vi "Configure Chart.vi"(8 "error in (no error)":errorcluster, 10 "Waveform Chart":refnum<vi>, 11 "Collection in":refnum<class "Collection.lvclass">) -> (0 "error out":errorcluster, 3 "Collection out":refnum<class "Collection.lvclass">)   [LabVIEW 2017, in "Collection.lvclass"]
uses:
  Collection.lvclass
  C:/LabVIEW-programs-dev/Instruments/Utility Classes/Readable/Readable.lvclass
  Readable/Readable.lvclass
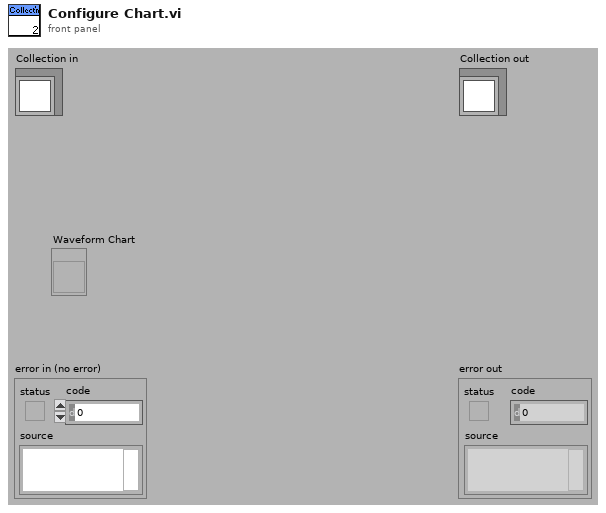
[diagram p1: front panel]
types:
  T1 = typedef "Readable.lvclass/Channel Names.ctl" = string[]
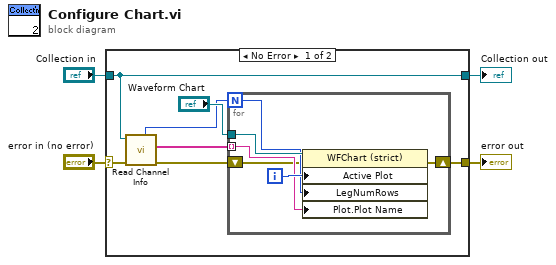
[diagram p0: block diagram]
diagram:
  n1 = case shown="No Error" "error in (no error)" {
    selector: "error in (no error)" -> [w8 w19]
    tunnel: [w10 w19] -> w3
    tunnel: [w9 w18] -> w1
    tunnel: "Collection in" -> [w9 w18]
    frame No Error {
      n2 = call "Read Channel Info.vi"("error in (no error)"=w8, "Readable.lvclass in"=w9) -> ("error out"=w7:errorcluster, "Channel Names"=w5:T1, "#Channels"=w6:i32)  [unwired: 5 in, 2 out]
      n3 = for {
        N: w6 -> [w14]
        tunnel: "Waveform Chart" -> [w17]
        shift-right: [w16] -> w10
        shift-left: w7 -> [w12]
        tunnel: w5 -> [w13] mode=indexing
        i -> [w15]
        n4 = property class="WFChart (strict)"(reference=w17, error in=w12, "Active Plot"=w15, "LegNumRows"=w14, "Plot.Plot Name"=w13) -> (error out=w16:errorcluster)  [unwired: 1 out]
      }
    }
    frame Error {
    }
  }
  "error out" <- w3
  "Collection out" <- w1
